vi "Draw Curve.vi"(8 "error in (no error)":errorcluster, 10 "Curve Extraction":T1, 11 "Refnum in":T2) -> (0 "error out":errorcluster, 3 "Refnum out":T2)   [LabVIEW 2019]
uses:
  <vilib>/vision/Image Controls.llb/IMAQ Image.ctl
  <vilib>/vision/NI_Vision_Development_Module.lvlib
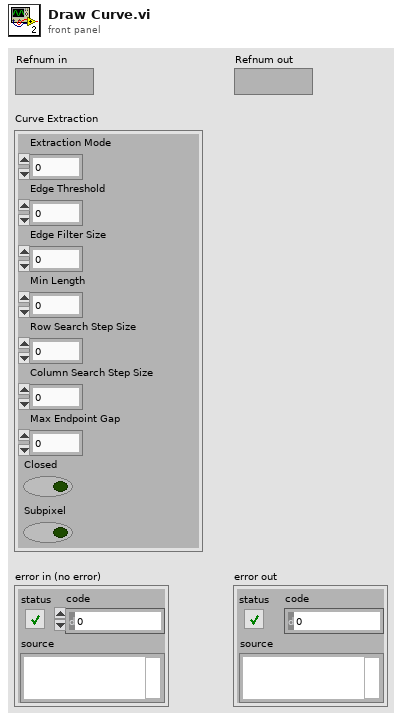
[diagram p1: front panel]
types:
  T1 = cluster{"Extraction Mode":u32, "Edge Threshold":i32, "Edge Filter Size":u32, "Min Length":i32, "Row Search Step Size":i32, "Column Search Step Size":i32, "Max Endpoint Gap":i32, "Closed":bool, "Subpixel":bool}
  T2 = typedef "IMAQ Image.ctl" = refnum<image>
  T3 = typedef "IMAQ ExtractCurvesCurve.ctl" = cluster{"Points":cluster{"X":dbl, "Y":dbl}[], "Closed?":bool, "Curve Length":dbl, "Min Edge Strength":dbl, "Max Edge Strength":dbl, "Average Edge Strength":dbl}
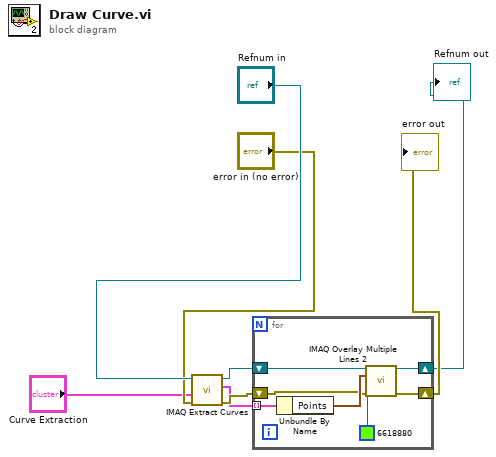
[diagram p0: block diagram]
diagram:
  n1 = call "IMAQ Extract Curves"("error in (no error)"="error in (no error)", "Curve Parameters"="Curve Extraction", "Image"="Refnum in") -> ("error out"=w5:errorcluster, "Curves"=w2:T3[], "Image (dup)"=w3:T2)  [unwired: 6 in]
  n2 = for {
    tunnel: w2 -> [w13] mode=indexing
    shift-right: [w11] -> w6
    shift-left: w3 -> [w12]
    shift-right: [w9] -> w7
    shift-left: w5 -> [w10]
    n3 = Unbundle By Name(w13) -> ("Points"=w15:cluster{"X":dbl, "Y":dbl}[])
    n4 = call "IMAQ Overlay Multiple Lines 2"("Image"=w12, "Line End Points"=w15, "Color"=u32 6618880, "error in (no error)"=w10) -> ("Image Out"=w11:T2, "error out"=w9:errorcluster)  [unwired: 10 in]
  }
  "error out" <- w7
  "Refnum out" <- w6
